vi "Statusword Auflösung.vi"() -> ()   [LabVIEW 2014]
panel:
  in  "Wert":u32 format="%x"
  out "13 Referenzfahrtfehler":bool
  out "12 Referenzfahrt durchgeführt":bool
  out "11 internal_limit_active":bool
  out "10 target_reached":bool
  out "9 remote (kann kommunizieren)":bool
  out "8":bool
  out "7 warning":bool
  out "6 switch on disable":bool
  out "5 quick stop":bool
  out "4 voltage enabled":bool
  out "3 fault":bool
  out "2 operation enable":bool
  out "1 switched on":bool
  out "0 ready to switch on":bool
  # "Auflösung des statuswords, Objekt 6041h S. 59 Kollmorgen S706 CanOpen Handbuch"
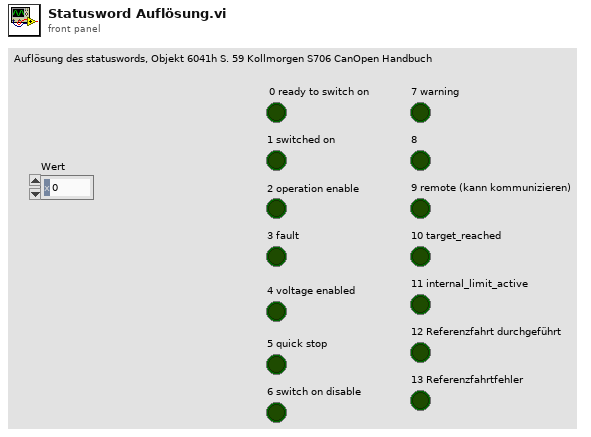
[diagram p1: front panel]
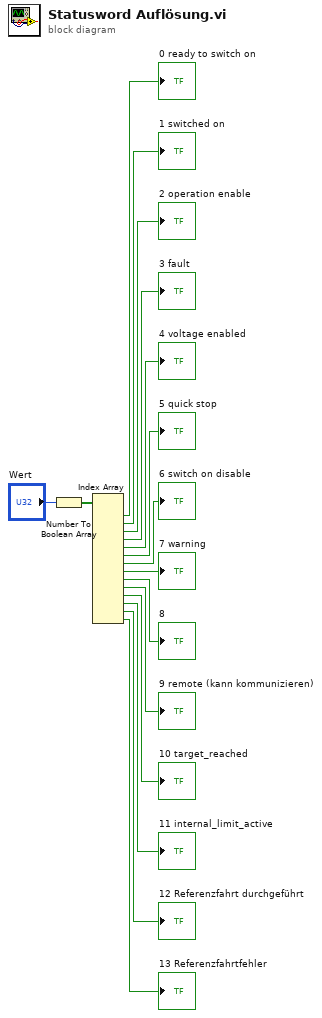
[diagram p0: block diagram]
diagram:
  n1 = Number To Boolean Array(number="Wert") -> (Boolean array=w15:bool[])
  n2 = Index Array(array=w15) -> (element #1=→"0 ready to switch on":bool, element #2=→"1 switched on":bool, element #3=→"2 operation enable":bool, element #4=→"3 fault":bool, element #5=→"4 voltage enabled":bool, element #6=→"5 quick stop":bool, element #7=→"6 switch on disable":bool, element #8=→"7 warning":bool, element #9=→"8":bool, element #10=→"9 remote (kann kommunizieren)":bool, element #11=→"10 target_reached":bool, element #12=→"11 internal_limit_active":bool, element #13=→"12 Referenzfahrt durchgeführt":bool, element #14=→"13 Referenzfahrtfehler":bool)  [unwired: 14 in]
